vi "DPT Panel Color Set.vi"(1 "TC Min OK Val":dbl, 2 "TC Max OK Val":dbl, 3 "StDev Thresh":dbl, 4 "Panel 1":T1[][](array[typedef])) -> (0 "Panel Out":T1[][](array[typedef]))   [LabVIEW 2014]
uses:
  Drivers/cDAQ/Type Definitions/cDAQ Sensor.ctl
panel:
  out "output cluster":T1={"Mean"=0.0, " Std"=0.0, "Color Box"=8585007}
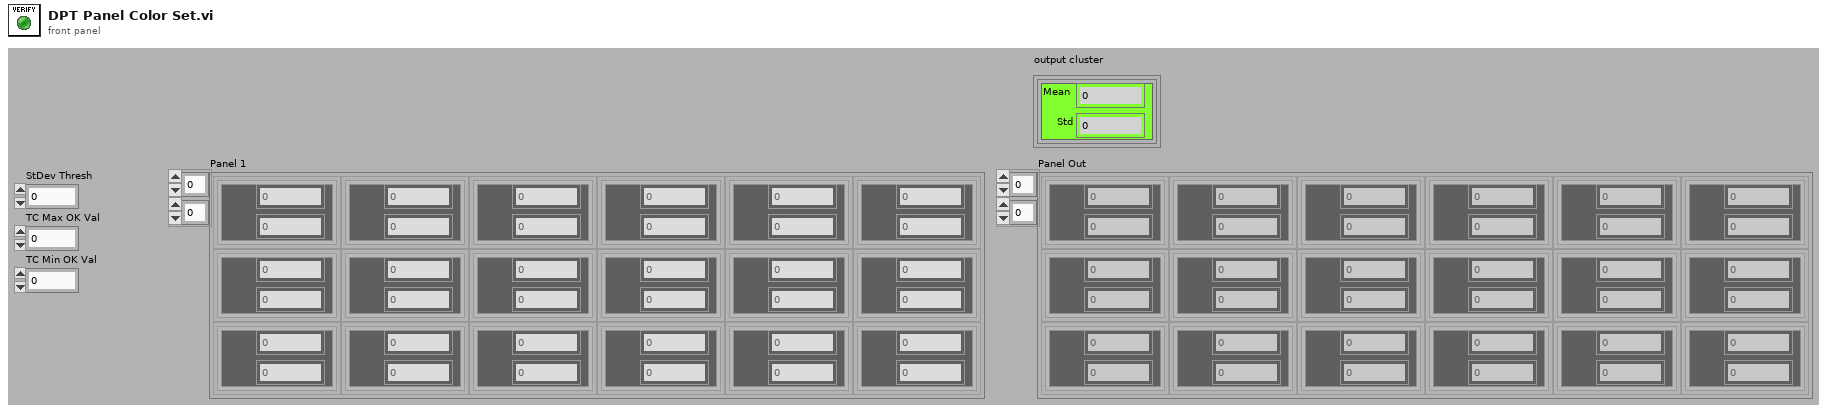
[diagram p1: front panel]
types:
  T1 = typedef "cDAQ Sensor.ctl" = cluster{"Mean":dbl, " Std":dbl, "Color Box":u32}
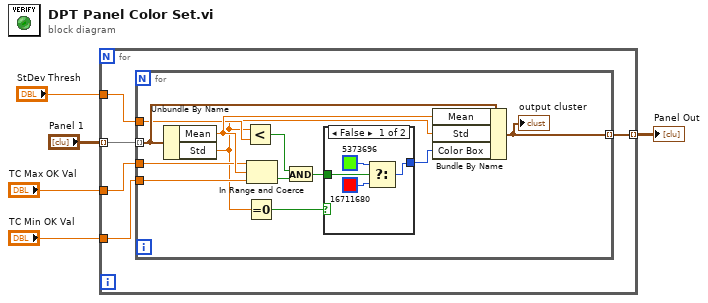
[diagram p0: block diagram]
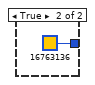
[diagram p2: hidden frame]
diagram:
  n1 = for {
    tunnel: [w10] -> w1 mode=indexing
    tunnel: "Panel 1" -> [w9] mode=indexing
    tunnel: "TC Max OK Val" -> [w8]
    tunnel: "TC Min OK Val" -> [w7]
    tunnel: "StDev Thresh" -> [w6]
    n2 = for {
      tunnel: [w22] -> w10 mode=indexing
      tunnel: w9 -> [w19] mode=indexing
      tunnel: w8 -> [w16]
      tunnel: w7 -> [w15]
      tunnel: w6 -> [w14]
      n3 = Unbundle By Name(w19) -> ("Mean"=w18:dbl, "Std"=w12:dbl)
      n4 = Less?(x=w12, y=w14) -> (x < y?=w21:bool)
      n5 = Equal To 0?(x=w12) -> (x = 0?=w11:bool)
      n6 = In Range and Coerce(upper limit=w16, x=w18, lower limit=w15) -> (In Range?=w17:bool)  [unwired: 1 out]
      n7 = And(x=w21, y=w17) -> (x .and. y?=w20:bool)
      n8 = case shown="False" w11 {
        tunnel: [w24 u32 16763136 ("Color Box")] -> w13
        tunnel: w20 -> [w23 _]
        frame False {
          n9 = Select(t=u32 5373696 ("Color Box"), s=w23, f=u32 16711680 ("Color Box")) -> (s? t:f=w24:u32)
        }
        frame True {
        }
      }
      n10 = Bundle By Name(cluster=w19, "Mean"=w18, "Std"=w12, "Color Box"=w13) -> (w22:T1)
      "output cluster" <- w22
    }
  }
  "Panel Out" <- w1
